vi "Show Profiles.vi"(8 "error in (no error)":errorcluster) -> (0 "error out":errorcluster, 3 "Feedback":string)   [LabVIEW 2012]
doc: "Displays a list of wireless profiles that are configured on the computer."
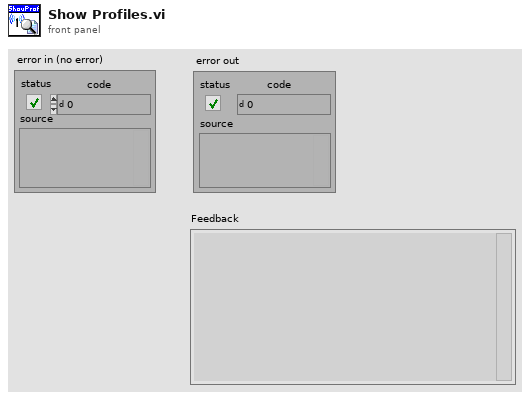
[diagram p1: front panel]
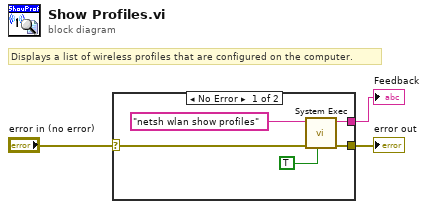
[diagram p0: block diagram]
diagram:
  # "Displays a list of wireless profiles that are configured on the computer."
  n1 = case shown="No Error" "error in (no error)" {
    selector: "error in (no error)" -> [w4 w9]
    tunnel: [w7 _] -> w3
    tunnel: [w5 w9] -> w2
    frame No Error {
      n2 = call <vilib>:"System Exec.vi"("run minimized? (F)"=TRUE, "error in (no error)"=w4, "command line"="netsh wlan show profiles") -> ("error out"=w5:errorcluster, "standard output"=w7:string)  [unwired: 5 in, 2 out]
    }
    frame Error {
    }
  }
  "Feedback" <- w3
  "error out" <- w2
